vi "WriteClassAttribute.vi"(5 "error in (no error)":errorcluster) -> (19 "error out":errorcluster)   [LabVIEW 2017, in "G#MethodTemplates.lvclass"]
uses:
  <vilib>/addons/_AddQ/G#Templates/G#MethodTemplates/G#MethodTemplates.lvclass
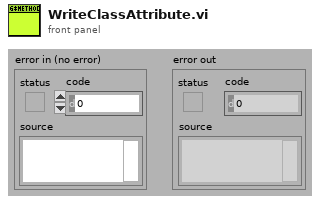
[diagram p1: front panel]
types:
  T1 = typedef "G#MethodTemplates.lvclass/ClassAttributesRef.ctl" = refnum<data-value>
  T2 = typedef "G#MethodTemplates.lvclass/ClassAttributes.ctl" = cluster{"Dummy":bool}
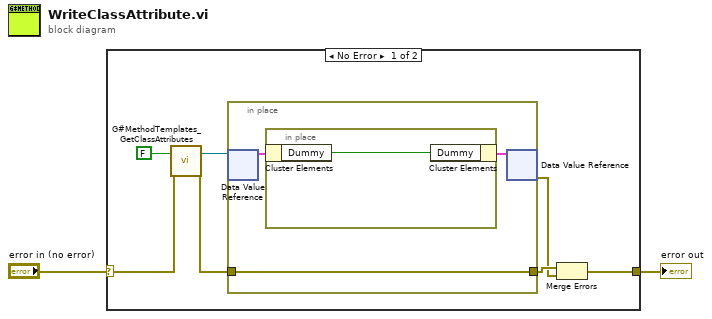
[diagram p0: block diagram]
diagram:
  n1 = case shown="No Error" "error in (no error)" {
    selector: "error in (no error)" -> [w9 w14]
    tunnel: [w6 w14] -> w1
    frame No Error {
      n2 = call <vilib>:"G#MethodTemplates_GetClassAttributes.vi"("return data? (T)"=FALSE ("return data"), "error in (no error)"=w9) -> ("class attributes ref"=w7:T1, "error out"=w8:errorcluster)  [unwired: 14 in, 2 out]
      n3 = in-place {
        in-place-border: w8 -> [w10]
        in-place-border: [w10] -> w4
        n4 = in-place-dvr #1(w7) -> (w11:T2)  [unwired: 1 out]
        n5 = in-place {
          n6 = in-place-cluster #2(w11) -> ("Dummy"=w13:bool)
          n7 = in-place-cluster #2("Dummy"=w13) -> (w12:T2)
        }
        n8 = in-place-dvr #1(w12) -> (w3:errorcluster)  [unwired: 1 out]
      }
      n9 = Merge Errors(w4, w3) -> (w6:errorcluster)
    }
    frame Error {
    }
  }
  "error out" <- w1
